vi "Update Data.vi"(8 "error in (no error)":errorcluster, 10 "Data Point":dbl, 11 "TXT Report in":refnum<class "TXT Report.lvclass">) -> (0 "error out":errorcluster, 3 "TXT Report out":refnum<class "TXT Report.lvclass">)   [LabVIEW 2009, in "TXT Report.lvclass"]
doc: "This dynamic dispatch VI updates data in a file for a TXT Report object.\n\nAAL 9/09"
uses:
  TXT Report.lvclass
  Report Class/Report.lvclass
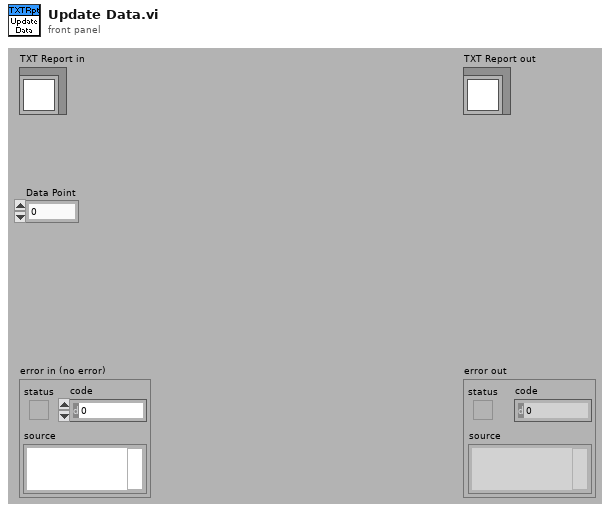
[diagram p1: front panel]
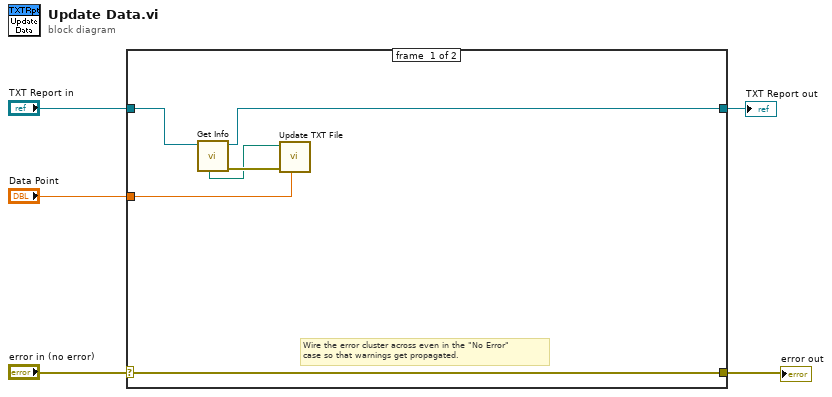
[diagram p0: block diagram]
diagram:
  n1 = case shown="No Error" "error in (no error)" {
    selector: "error in (no error)" -> [w11 w13]
    tunnel: [w11 w13] -> w1
    tunnel: [w7 w12] -> w2
    tunnel: "TXT Report in" -> [w8 w12]
    tunnel: "Data Point" -> [w6 _]
    frame #0 {
      # "Wire the error cluster across even in the \"No Error\"\ncase so that warnings get propagated."
      n2 = call "Get Info.vi"("Report"=w8) -> ("error out"=w10:errorcluster, "Report out"=w7:refnum<class "TXT Report.lvclass">, "Path"=w9:path)  [unwired: 1 in, 7 out]
      n3 = call "Update TXT File.vi"("Data Point"=w6, "error in"=w10, "Path"=w9) -> ()  [unwired: 8 in, 1 out]
    }
    frame #1 {
    }
  }
  "error out" <- w1
  "TXT Report out" <- w2
